vi "ClusterEscala.vi.vi"() -> ()   [LabVIEW 2020]
panel:
  out "Indicador":cluster{dbl, dbl, dbl} {"?" scale=0.0..10.0; "?" scale=0.0..100.0; "?" scale=0.0..100.0}
  in  "Cluster":T1
  # "V (flujo)"
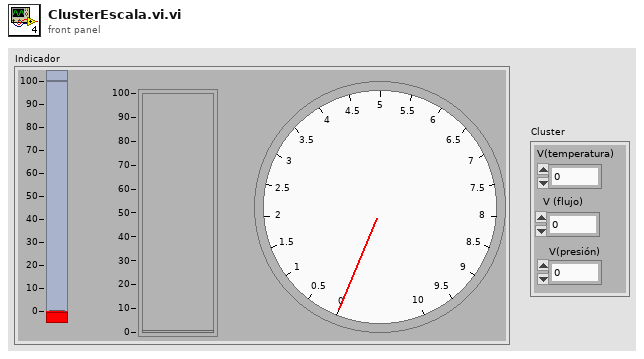
[diagram p1: front panel]
types:
  T1 = cluster{"V(temperatura)":dbl, dbl, "V(presión)":dbl}
  T2 = cluster{"(I/seg)/V":dbl, "(N/m^2)/V":dbl, "°C/V":dbl}
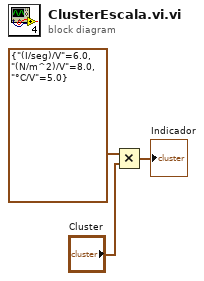
[diagram p0: block diagram]
diagram:
  n1 = Multiply(x=T2 {"(I/seg)/V"=6.0, "(N/m^2)/V"=8.0, "°C/V"=5.0}, y="Cluster") -> (x*y=→"Indicador":cluster{dbl, dbl, dbl})
